vi "to string.vi"(8 "error in":errorcluster, 11 "Standard Engine Repo Data in":refnum<class "Standard Engine Configuration.lvclass">) -> (0 "error out":errorcluster, 1 "data":string, 2 "version":string, 3 "Standard Engine Repo Data out":refnum<class "Standard Engine Configuration.lvclass">)   [LabVIEW 2013, in "Standard Engine Configuration.lvclass"]
uses:
  Standard Engine Configuration.lvclass
  <vilib>/NI/Module Execution Interface/Engine Configuration/engine configuration.lvclass
  Standard Engine Configuration.lvclass/Standard Engine Configuration.ctl
  <vilib>/NI/Configuration Framework/serializable configuration/NISE_CEF_serializable configuration.lvclass
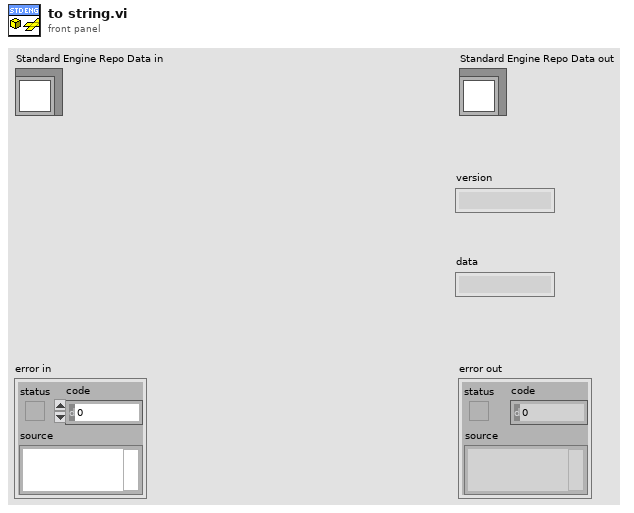
[diagram p1: front panel]
types:
  T1 = typedef "Standard Engine Configuration.lvclass/Module Specific Configuration.ctl" = cluster{"Module ID":string, "Module Decimation":T2, "error tag":string, "error responses":T3, "Initialize on Error?":bool}
  T2 = typedef "Standard Engine Configuration.lvclass/Module Decimation.ctl" = cluster{"Decimation":u16, "Offset":u16, "sort order":i32, "async?":bool}
  T3 = typedef "Standard Engine Configuration.lvclass/error responses.ctl" = cluster{"unknown":T4, "trivial":T4, "critical":T4, "recoverable":T4}
  T4 = typedef "Standard Engine Configuration.lvclass/error options.ctl" = cluster{"clear":bool, "notify":bool, "log":bool, "remove module":bool, "abort engine":bool, "go to safe state":bool, "recover module":bool}
  T5 = typedef "Standard Engine Configuration.lvclass/Loop Info.ctl" = cluster{"Processor":i32, "Priority":i32, "timing source type":T6, "module providing source":string, "timing source dt":u32, "timing policy":T7}
  T6 = typedef "Standard Engine Configuration.lvclass/Supported Timing Sources.ctl" = enum16{"Use Module Timing Source", "1 kHz Clock", "1 MHz Clock", "Synchronize to Scan Engine"}
  T7 = typedef "Standard Engine Configuration.lvclass/timing policy.ctl" = enum16{"strict determinism", "nonblocking", "nondeterministic inline"}
  T8 = typedef "Standard Engine Configuration.lvclass/execution timing tags.ctl" = cluster{"iteration start time (DBL)":string, "inputs duration (DBL)":string, "process duration (DBL)":string, "outputs duration (DBL)":string}
  T9 = cluster{"unknown.log":bool, "trivial.log":bool, "critical.log":bool, "recovereable.log":bool}[]
  T10 = cluster{"Module ID":string, "Module Decimation":T2, "error tag":string, "error responses":cluster{"unknown":cluster{"clear":bool, "notify":bool, "remove module":bool, "abort engine":bool, "go to safe state":bool, "recover module":bool}, "trivial":cluster{"clear":bool, "notify":bool, "remove module":bool, "abort engine":bool, "go to safe state":bool, "recover module":bool}, "critical":cluster{"clear":bool, "notify":bool, "remove module":bool, "abort engine":bool, "go to safe state":bool, "recover module":bool}, "recoverable":cluster{"clear":bool, "notify":bool, "remove module":bool, "abort engine":bool, "go to safe state":bool, "recover module":bool}}, "Initialize on Error?":bool}[]
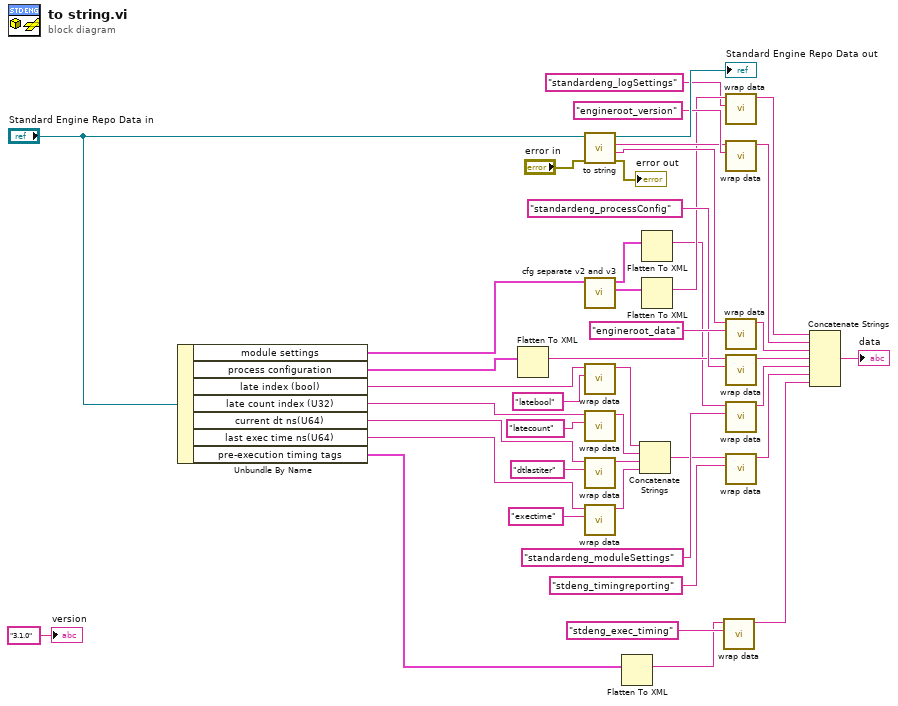
[diagram p0: block diagram]
diagram:
  n1 = Unbundle By Name("Standard Engine Repo Data in") -> ("module settings"=w11:T1[], "process configuration"=w30:T5, "late index (bool)"=w26:string, "late count index (U32)"=w25:string, "current dt ns(U64)"=w24:string, "last exec time ns(U64)"=w12:string, "pre-execution timing tags"=w3:T8)
  n2 = Flatten To XML(anything=w30) -> (xml string=w31:string)
  n3 = call-parent "to string.vi"("error in"="error in", "engine configuration in"="Standard Engine Repo Data in") -> ("error out"=→"error out":errorcluster, "data"=w33:string, "version"=w34:string, "engine configuration out"=→"Standard Engine Repo Data out":refnum<class "Standard Engine Configuration.lvclass">)  [unwired: 6 in]
  n4 = call "cfg separate v2 and v3.vi"("Engine Configuration In"=w11) -> ("Log Actions"=w9:T9, "Engine Configuration Out"=w10:T10)  [unwired: 8 in, 1 out]
  n5 = call <vilib>:"wrap data.vi"("identifier"="latebool", "data to wrap"=w26) -> ("wrapped data"=w21:string)  [unwired: 9 in]
  n6 = call <vilib>:"wrap data.vi"("identifier"="latecount", "data to wrap"=w25) -> ("wrapped data"=w22:string)  [unwired: 9 in]
  n7 = call <vilib>:"wrap data.vi"("identifier"="dtlastiter", "data to wrap"=w24) -> ("wrapped data"=w23:string)  [unwired: 9 in]
  n8 = call <vilib>:"wrap data.vi"("identifier"="exectime", "data to wrap"=w12) -> ("wrapped data"=w13:string)  [unwired: 9 in]
  n9 = Flatten To XML(anything=w3) -> (xml string=w2:string)
  n10 = Concatenate Strings(w21, w22, w23, w13) -> (w20:string)
  n11 = Flatten To XML(anything=w10) -> (xml string=w1:string)
  n12 = Flatten To XML(anything=w9) -> (xml string=w8:string)
  n13 = call <vilib>:"wrap data.vi"("identifier"="stdeng_exec_timing", "data to wrap"=w2) -> ("wrapped data"=w4:string)  [unwired: 9 in]
  n14 = call <vilib>:"wrap data.vi"("identifier"="standardeng_logSettings", "data to wrap"=w8) -> ("wrapped data"=w6:string)  [unwired: 9 in]
  n15 = call <vilib>:"wrap data.vi"("identifier"="engineroot_version" ("additional identifier"), "data to wrap"=w34) -> ("wrapped data"=w37:string)  [unwired: 9 in]
  n16 = call <vilib>:"wrap data.vi"("identifier"="engineroot_data" ("additional identifier"), "data to wrap"=w33) -> ("wrapped data"=w38:string)  [unwired: 9 in]
  n17 = call <vilib>:"wrap data.vi"("identifier"="standardeng_processConfig" ("additional identifier"), "data to wrap"=w31) -> ("wrapped data"=w35:string)  [unwired: 9 in]
  n18 = call <vilib>:"wrap data.vi"("identifier"="standardeng_moduleSettings" ("additional identifier"), "data to wrap"=w1) -> ("wrapped data"=w28:string)  [unwired: 9 in]
  n19 = call <vilib>:"wrap data.vi"("identifier"="stdeng_timingreporting", "data to wrap"=w20) -> ("wrapped data"=w18:string)  [unwired: 9 in]
  n20 = Concatenate Strings(w6, w37, w38, w35, w28, w18, w4) -> (→"data":string)
  "version" <- "3.1.0" ("Version")
